vi "2_4_Operaciones.vi"() -> ()   [LabVIEW 2020]
panel:
  in  "?":bool
  out "?":string
  in  "?":bool
  in  "?":bool
  in  "?":bool
  in  "?":bool
  in  "B":dbl
  in  "A":dbl
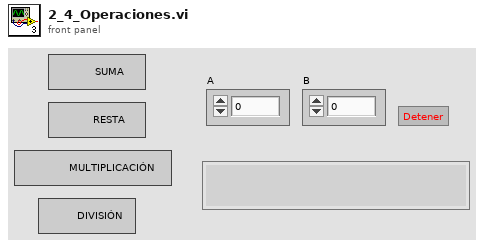
[diagram p1: front panel]
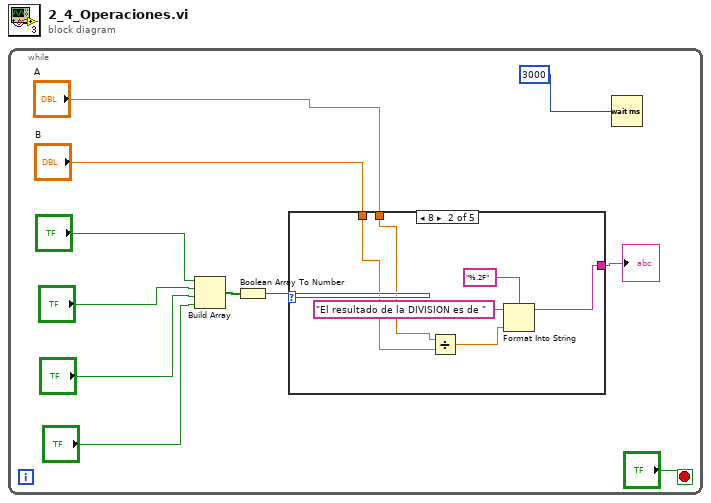
[diagram p0: block diagram]
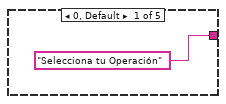
[diagram p2: hidden frame]
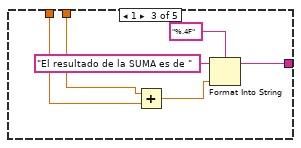
[diagram p3: hidden frame]
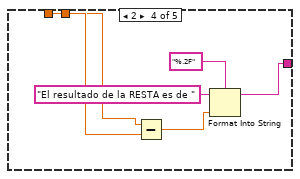
[diagram p4: hidden frame]
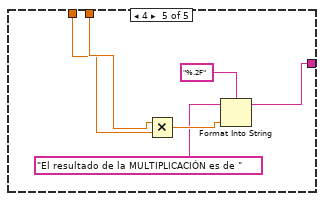
[diagram p5: hidden frame]
diagram:
  n1 = while {
    stop <- "?" stop-if-true
    n2 = Build Array("?", "?", "?", "?") -> (w7:bool[])
    n3 = Boolean Array To Number(Boolean array=w7) -> (number=w6:u32)
    n4 = case shown="8" w6 {
      tunnel: "A" -> [_ w14 w24 w25 w33]
      tunnel: "B" -> [_ w13 w23 w26 w32]
      tunnel: ["Selecciona tu Operación" w15 w19 w27 w31] -> w3
      frame 0, Default {
      }
      frame 8 {
        n5 = Divide(x=w14, y=w13) -> (x/y=w18:dbl)
        n6 = Format Into String(format string="%.2F", initial string="El resultado de la DIVISION es de ", w18) -> (resulting string=w15:string)  [unwired: 1 in, 1 out]
      }
      frame 1 {
        n7 = Add(x=w24, y=w23) -> (x+y=w22:dbl)
        n8 = Format Into String(format string="%.4F", initial string="El resultado de la SUMA es de ", w22) -> (resulting string=w19:string)  [unwired: 1 in, 1 out]
      }
      frame 2 {
        n9 = Subtract(x=w25, y=w26) -> (x-y=w30:dbl)
        n10 = Format Into String(format string="%.2F", initial string="El resultado de la RESTA es de ", w30) -> (resulting string=w27:string)  [unwired: 1 in, 1 out]
      }
      frame 4 {
        n11 = Multiply(x=w33, y=w32) -> (x*y=w36:dbl)
        n12 = Format Into String(format string="%.2F", initial string="El resultado de la MULTIPLICACIÓN es de ", w36) -> (resulting string=w31:string)  [unwired: 1 in, 1 out]
      }
    }
    "?" <- w3
    n13 = Wait (ms)(milliseconds to wait=3000) -> ()  [unwired: 1 out]
  }
